vi "LHPulse-10-06-17.vi"(1 "LHPulse(us)":T1, 2 "LHHeizen2?":T2, 3 "LHHeizen1?":T2) -> ()   [LabVIEW 2010]
uses:
  <vilib>/eio/EIONode/EIONode.xnode
  <vilib>/rvi/eio/nirviEIOImplementation/nirviEIOImplementation.xnode
  <vilib>/rvi/eio/common/nirviEmuClasses.ctl
  <vilib>/rvi/eio/common/nirviEmuTemplateMethod_noerrors.vi
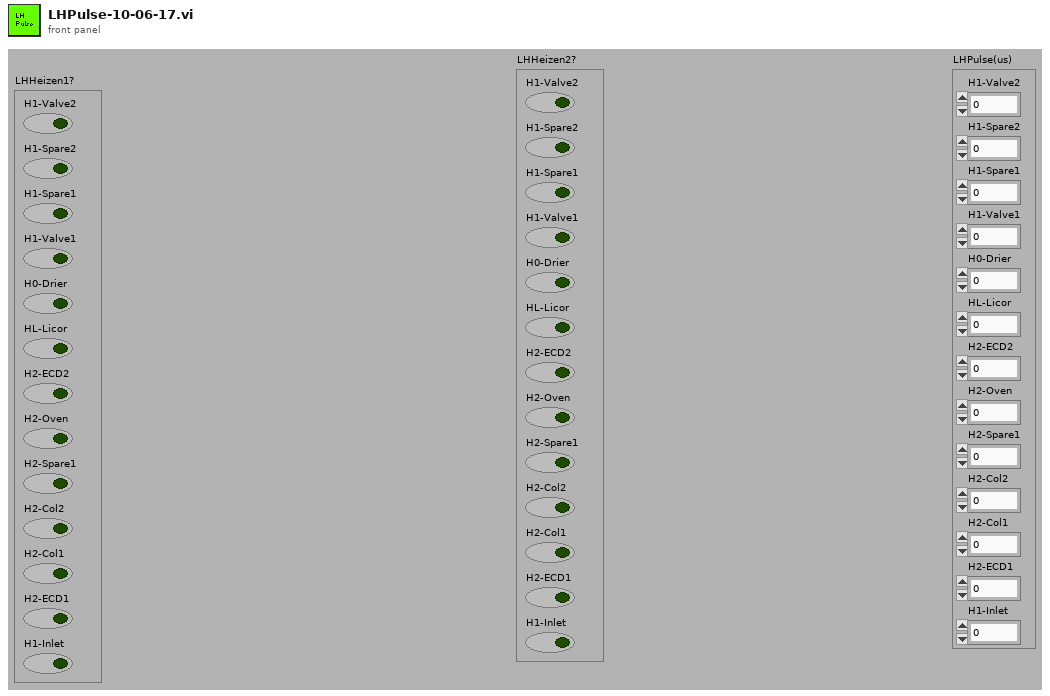
[diagram p1: front panel]
types:
  T1 = cluster{"H1-Valve2":u32, "H1-Spare2":u32, "H1-Spare1":u32, "H1-Valve1":u32, "H0-Drier":u32, "HL-Licor":u32, "H2-ECD2":u32, "H2-Oven":u32, "H2-Spare1":u32, "H2-Col2":u32, "H2-Col1":u32, "H2-ECD1":u32, "H1-Inlet":u32}
  T2 = cluster{"H1-Valve2":bool, "H1-Spare2":bool, "H1-Spare1":bool, "H1-Valve1":bool, "H0-Drier":bool, "HL-Licor":bool, "H2-ECD2":bool, "H2-Oven":bool, "H2-Spare1":bool, "H2-Col2":bool, "H2-Col1":bool, "H2-ECD1":bool, "H1-Inlet":bool}
  T3 = typedef "nirviEmuClasses.ctl" = enum16{"IO Read", "IO Write", "Method", "Property Read", "Property Write"}
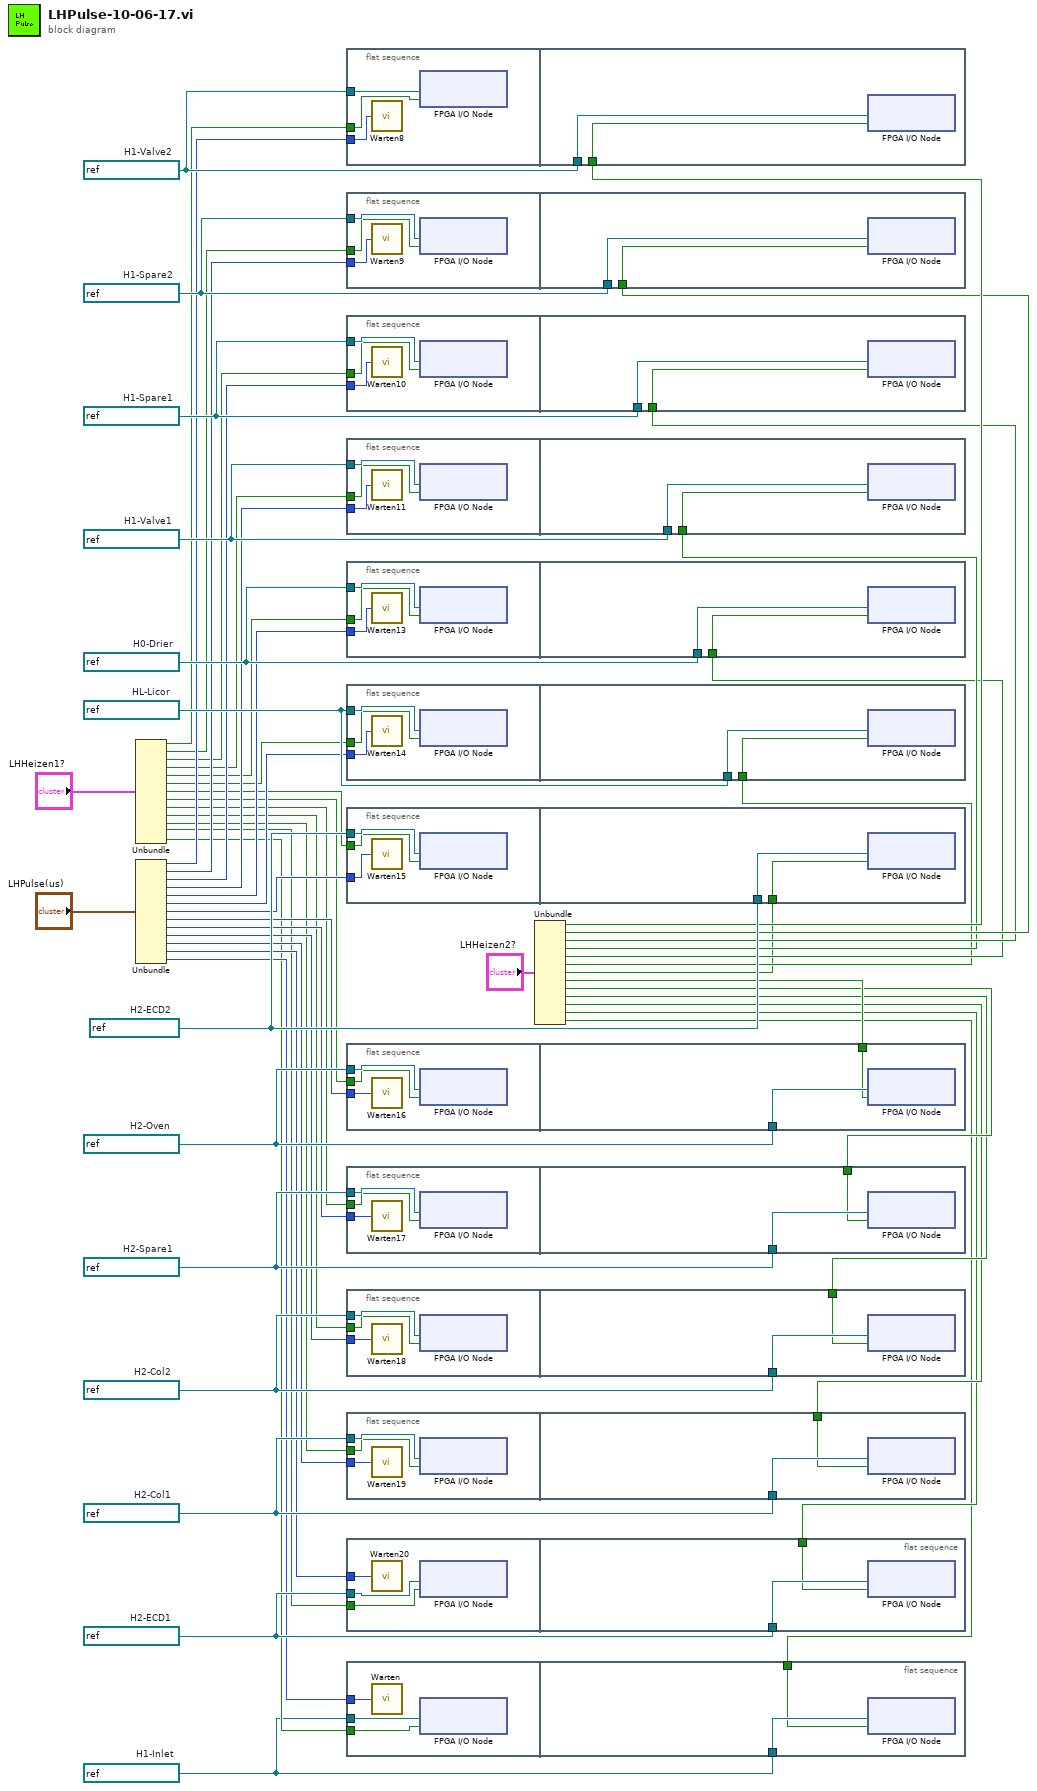
[diagram p0: block diagram]
diagram:
  w1 = refnum<k21> "Mod5/DIO14"  # H1-Inlet
  w44 = refnum<k21> "Mod5/DIO20"  # H2-ECD1
  w45 = refnum<k21> "Mod5/DIO19"  # H2-Col1
  w46 = refnum<k21> "Mod5/DIO18"  # H2-Col2
  w47 = refnum<k21> "Mod5/DIO17"  # H2-Spare1
  w48 = refnum<k21> "Mod5/DIO16"  # H2-Oven
  w49 = refnum<k21> "Mod5/DIO1"  # H2-ECD2
  w50 = refnum<k21> "Mod5/DIO27"  # HL-Licor
  w51 = refnum<k21> "Mod5/DIO31"  # H0-Drier
  w52 = refnum<k21> "Mod6/DIO27"  # H1-Valve1
  w53 = refnum<k21> "Mod6/DIO26"  # H1-Spare1
  w54 = refnum<k21> "Mod6/DIO25"  # H1-Spare2
  w55 = refnum<k21> "Mod6/DIO24"  # H1-Valve2
  n1 = Unbundle("LHHeizen1?") -> ("H1-Valve2"=w31:bool, "H1-Spare2"=w30:bool, "H1-Spare1"=w29:bool, "H1-Valve1"=w28:bool, "H0-Drier"=w27:bool, "HL-Licor"=w26:bool, "H2-ECD2"=w25:bool, "H2-Oven"=w24:bool, "H2-Spare1"=w23:bool, "H2-Col2"=w22:bool, "H2-Col1"=w21:bool, "H2-ECD1"=w20:bool, "H1-Inlet"=w3:bool)
  n2 = Unbundle("LHPulse(us)") -> ("H1-Valve2"=w43:u32, "H1-Spare2"=w42:u32, "H1-Spare1"=w41:u32, "H1-Valve1"=w40:u32, "H0-Drier"=w39:u32, "HL-Licor"=w38:u32, "H2-ECD2"=w37:u32, "H2-Oven"=w36:u32, "H2-Spare1"=w35:u32, "H2-Col2"=w34:u32, "H2-Col1"=w33:u32, "H2-ECD1"=w32:u32, "H1-Inlet"=w4:u32)
  n3 = flat-sequence {
    tunnel: w55 -> [w58]
    tunnel: w31 -> [w57]
    tunnel: w43 -> [w56]
    tunnel: w55 -> [w71]
    tunnel: w19 -> [w70]
    frame #0 {
      n4 = call "Warten8"("Count(uSec)"=w56) -> ()  [unwired: 1 out]
      n5 = xnode "FPGA I/O Node"("I/O Item"=w57, "FPGA I/O In"=w58) -> ()  [unwired: 1 out]
    }
    frame #1 {
      n6 = xnode "FPGA I/O Node"("I/O Item"=w70, "FPGA I/O In"=w71) -> ()  [unwired: 1 out]
    }
  }
  n7 = flat-sequence {
    tunnel: w54 -> [w85]
    tunnel: w30 -> [w84]
    tunnel: w42 -> [w83]
    tunnel: w54 -> [w98]
    tunnel: w18 -> [w97]
    frame #0 {
      n8 = call "Warten9"("Count(uSec)"=w83) -> ()  [unwired: 1 out]
      n9 = xnode "FPGA I/O Node"("I/O Item"=w84, "FPGA I/O In"=w85) -> ()  [unwired: 1 out]
    }
    frame #1 {
      n10 = xnode "FPGA I/O Node"("I/O Item"=w97, "FPGA I/O In"=w98) -> ()  [unwired: 1 out]
    }
  }
  n11 = flat-sequence {
    tunnel: w53 -> [w112]
    tunnel: w29 -> [w111]
    tunnel: w41 -> [w110]
    tunnel: w53 -> [w125]
    tunnel: w17 -> [w124]
    frame #0 {
      n12 = call "Warten10"("Count(uSec)"=w110) -> ()  [unwired: 1 out]
      n13 = xnode "FPGA I/O Node"("I/O Item"=w111, "FPGA I/O In"=w112) -> ()  [unwired: 1 out]
    }
    frame #1 {
      n14 = xnode "FPGA I/O Node"("I/O Item"=w124, "FPGA I/O In"=w125) -> ()  [unwired: 1 out]
    }
  }
  n15 = flat-sequence {
    tunnel: w52 -> [w139]
    tunnel: w28 -> [w138]
    tunnel: w40 -> [w137]
    tunnel: w52 -> [w152]
    tunnel: w16 -> [w151]
    frame #0 {
      n16 = call "Warten11"("Count(uSec)"=w137) -> ()  [unwired: 1 out]
      n17 = xnode "FPGA I/O Node"("I/O Item"=w138, "FPGA I/O In"=w139) -> ()  [unwired: 1 out]
    }
    frame #1 {
      n18 = xnode "FPGA I/O Node"("I/O Item"=w151, "FPGA I/O In"=w152) -> ()  [unwired: 1 out]
    }
  }
  n19 = flat-sequence {
    tunnel: w51 -> [w166]
    tunnel: w27 -> [w165]
    tunnel: w39 -> [w164]
    tunnel: w51 -> [w179]
    tunnel: w15 -> [w178]
    frame #0 {
      n20 = call "Warten13"("Count(uSec)"=w164) -> ()  [unwired: 1 out]
      n21 = xnode "FPGA I/O Node"("I/O Item"=w165, "FPGA I/O In"=w166) -> ()  [unwired: 1 out]
    }
    frame #1 {
      n22 = xnode "FPGA I/O Node"("I/O Item"=w178, "FPGA I/O In"=w179) -> ()  [unwired: 1 out]
    }
  }
  n23 = flat-sequence {
    tunnel: w50 -> [w193]
    tunnel: w26 -> [w192]
    tunnel: w38 -> [w191]
    tunnel: w50 -> [w206]
    tunnel: w14 -> [w205]
    frame #0 {
      n24 = call "Warten14"("Count(uSec)"=w191) -> ()  [unwired: 1 out]
      n25 = xnode "FPGA I/O Node"("I/O Item"=w192, "FPGA I/O In"=w193) -> ()  [unwired: 1 out]
    }
    frame #1 {
      n26 = xnode "FPGA I/O Node"("I/O Item"=w205, "FPGA I/O In"=w206) -> ()  [unwired: 1 out]
    }
  }
  n27 = flat-sequence {
    tunnel: w49 -> [w220]
    tunnel: w25 -> [w219]
    tunnel: w37 -> [w218]
    tunnel: w49 -> [w233]
    tunnel: w13 -> [w232]
    frame #0 {
      n28 = call "Warten15"("Count(uSec)"=w218) -> ()  [unwired: 1 out]
      n29 = xnode "FPGA I/O Node"("I/O Item"=w219, "FPGA I/O In"=w220) -> ()  [unwired: 1 out]
    }
    frame #1 {
      n30 = xnode "FPGA I/O Node"("I/O Item"=w232, "FPGA I/O In"=w233) -> ()  [unwired: 1 out]
    }
  }
  n31 = flat-sequence {
    tunnel: w48 -> [w247]
    tunnel: w24 -> [w246]
    tunnel: w36 -> [w245]
    tunnel: w48 -> [w260]
    tunnel: w12 -> [w259]
    frame #0 {
      n32 = call "Warten16"("Count(uSec)"=w245) -> ()  [unwired: 1 out]
      n33 = xnode "FPGA I/O Node"("I/O Item"=w246, "FPGA I/O In"=w247) -> ()  [unwired: 1 out]
    }
    frame #1 {
      n34 = xnode "FPGA I/O Node"("I/O Item"=w259, "FPGA I/O In"=w260) -> ()  [unwired: 1 out]
    }
  }
  n35 = flat-sequence {
    tunnel: w47 -> [w274]
    tunnel: w23 -> [w273]
    tunnel: w35 -> [w272]
    tunnel: w47 -> [w287]
    tunnel: w11 -> [w286]
    frame #0 {
      n36 = call "Warten17"("Count(uSec)"=w272) -> ()  [unwired: 1 out]
      n37 = xnode "FPGA I/O Node"("I/O Item"=w273, "FPGA I/O In"=w274) -> ()  [unwired: 1 out]
    }
    frame #1 {
      n38 = xnode "FPGA I/O Node"("I/O Item"=w286, "FPGA I/O In"=w287) -> ()  [unwired: 1 out]
    }
  }
  n39 = flat-sequence {
    tunnel: w46 -> [w301]
    tunnel: w22 -> [w300]
    tunnel: w34 -> [w299]
    tunnel: w46 -> [w314]
    tunnel: w10 -> [w313]
    frame #0 {
      n40 = call "Warten18"("Count(uSec)"=w299) -> ()  [unwired: 1 out]
      n41 = xnode "FPGA I/O Node"("I/O Item"=w300, "FPGA I/O In"=w301) -> ()  [unwired: 1 out]
    }
    frame #1 {
      n42 = xnode "FPGA I/O Node"("I/O Item"=w313, "FPGA I/O In"=w314) -> ()  [unwired: 1 out]
    }
  }
  n43 = flat-sequence {
    tunnel: w45 -> [w328]
    tunnel: w21 -> [w327]
    tunnel: w33 -> [w326]
    tunnel: w45 -> [w341]
    tunnel: w9 -> [w340]
    frame #0 {
      n44 = call "Warten19"("Count(uSec)"=w326) -> ()  [unwired: 1 out]
      n45 = xnode "FPGA I/O Node"("I/O Item"=w327, "FPGA I/O In"=w328) -> ()  [unwired: 1 out]
    }
    frame #1 {
      n46 = xnode "FPGA I/O Node"("I/O Item"=w340, "FPGA I/O In"=w341) -> ()  [unwired: 1 out]
    }
  }
  n47 = flat-sequence {
    tunnel: w44 -> [w355]
    tunnel: w20 -> [w354]
    tunnel: w32 -> [w353]
    tunnel: w44 -> [w368]
    tunnel: w8 -> [w367]
    frame #0 {
      n48 = call "Warten20"("Count(uSec)"=w353) -> ()  [unwired: 1 out]
      n49 = xnode "FPGA I/O Node"("I/O Item"=w354, "FPGA I/O In"=w355) -> ()  [unwired: 1 out]
    }
    frame #1 {
      n50 = xnode "FPGA I/O Node"("I/O Item"=w367, "FPGA I/O In"=w368) -> ()  [unwired: 1 out]
    }
  }
  n51 = flat-sequence {
    tunnel: w1 -> [w382]
    tunnel: w3 -> [w381]
    tunnel: w4 -> [w380]
    tunnel: w1 -> [w395]
    tunnel: w2 -> [w394]
    frame #0 {
      n52 = call "Warten"("Count(uSec)"=w380) -> ()  [unwired: 1 out]
      n53 = xnode "FPGA I/O Node"("I/O Item"=w381, "FPGA I/O In"=w382) -> ()  [unwired: 1 out]
    }
    frame #1 {
      n54 = xnode "FPGA I/O Node"("I/O Item"=w394, "FPGA I/O In"=w395) -> ()  [unwired: 1 out]
    }
  }
  n55 = Unbundle("LHHeizen2?") -> ("H1-Valve2"=w19:bool, "H1-Spare2"=w18:bool, "H1-Spare1"=w17:bool, "H1-Valve1"=w16:bool, "H0-Drier"=w15:bool, "HL-Licor"=w14:bool, "H2-ECD2"=w13:bool, "H2-Oven"=w12:bool, "H2-Spare1"=w11:bool, "H2-Col2"=w10:bool, "H2-Col1"=w9:bool, "H2-ECD1"=w8:bool, "H1-Inlet"=w2:bool)
